vi "set_frequency.vi"(8 "error in (no error)":errorcluster, 9 "Value 2":dbl, 10 "Value":string, 11 "VISA Refnum in":refnum<visa-resource-name>) -> (0 "error out":errorcluster, 3 "VISA Refnum out":refnum<visa-resource-name>)   [LabVIEW 2015]
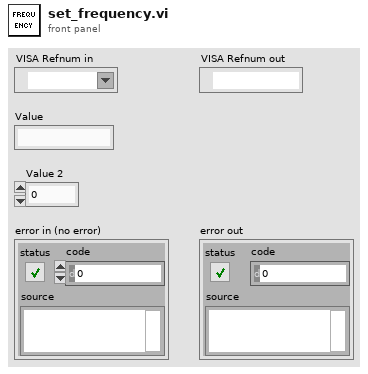
[diagram p1: front panel]
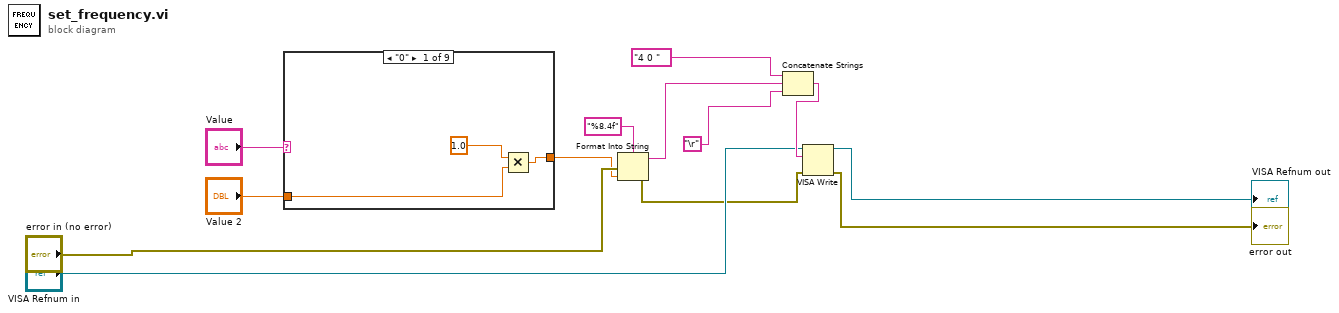
[diagram p0: block diagram]
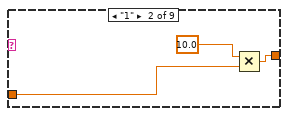
[diagram p2: hidden frame]
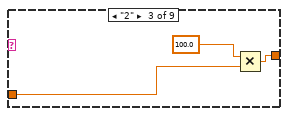
[diagram p3: hidden frame]
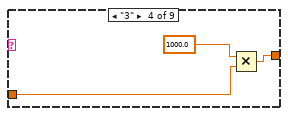
[diagram p4: hidden frame]
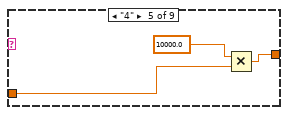
[diagram p5: hidden frame]
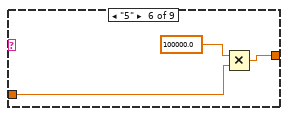
[diagram p6: hidden frame]
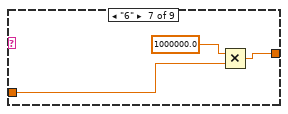
[diagram p7: hidden frame]
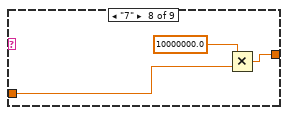
[diagram p8: hidden frame]
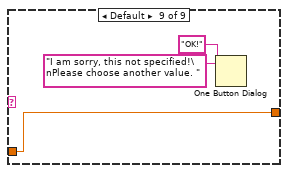
[diagram p9: hidden frame]
diagram:
  n1 = case shown="\"0\"" "Value" {
    tunnel: "Value 2" -> [w15 w18 w21 w24 w27 w30 w33 w36 w40]
    tunnel: [w14 w17 w20 w23 w26 w29 w32 w35 w40] -> w6
    frame "0" {
      n2 = Multiply(x=1.0 ("Frequency"), y=w15) -> (x*y=w14:dbl)
    }
    frame "1" {
      n3 = Multiply(x=10.0 ("Frequency"), y=w18) -> (x*y=w17:dbl)
    }
    frame "2" {
      n4 = Multiply(x=100.0 ("Frequency"), y=w21) -> (x*y=w20:dbl)
    }
    frame "3" {
      n5 = Multiply(x=1000.0 ("Frequency"), y=w24) -> (x*y=w23:dbl)
    }
    frame "4" {
      n6 = Multiply(x=10000.0 ("Frequency"), y=w27) -> (x*y=w26:dbl)
    }
    frame "5" {
      n7 = Multiply(x=100000.0 ("Frequency"), y=w30) -> (x*y=w29:dbl)
    }
    frame "6" {
      n8 = Multiply(x=1000000.0 ("Frequency"), y=w33) -> (x*y=w32:dbl)
    }
    frame "7" {
      n9 = Multiply(x=10000000.0 ("Frequency"), y=w36) -> (x*y=w35:dbl)
    }
    frame Default {
      n10 = One Button Dialog(message="I am sorry, this not specified!\nPlease choose another value. ", button name ("OK")="OK!") -> ()  [unwired: 1 out]
    }
  }
  n11 = Format Into String(format string="%8.4f", error in="error in (no error)", w6) -> (resulting string=w12:string, error out=w2:errorcluster)  [unwired: 1 in]
  n12 = Concatenate Strings("4 0 " ("string"), w12, "\r") -> (w13:string)
  n13 = VISA Write(VISA resource name="VISA Refnum in", write buffer=w13, error in (no error)=w2) -> (VISA resource name out=→"VISA Refnum out":refnum<visa-resource-name>, error out=→"error out":errorcluster)  [unwired: 1 out]
